vi "Jeffress_model_v004.vi"() -> ()   [LabVIEW 2019]
panel:
  out "Index":string
  out "new picture":picture
  in  "stop":bool
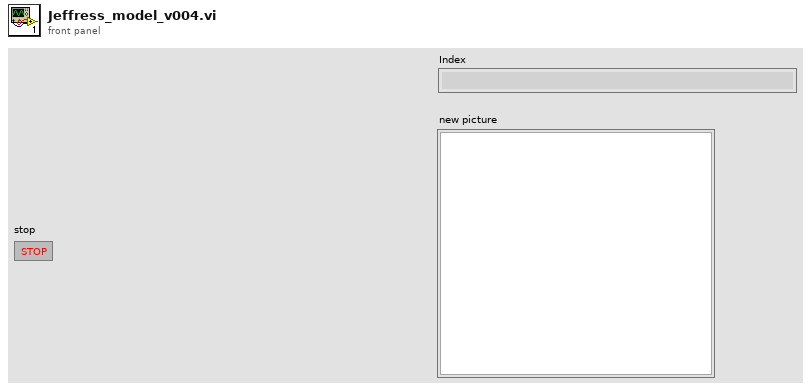
[diagram p1: front panel]
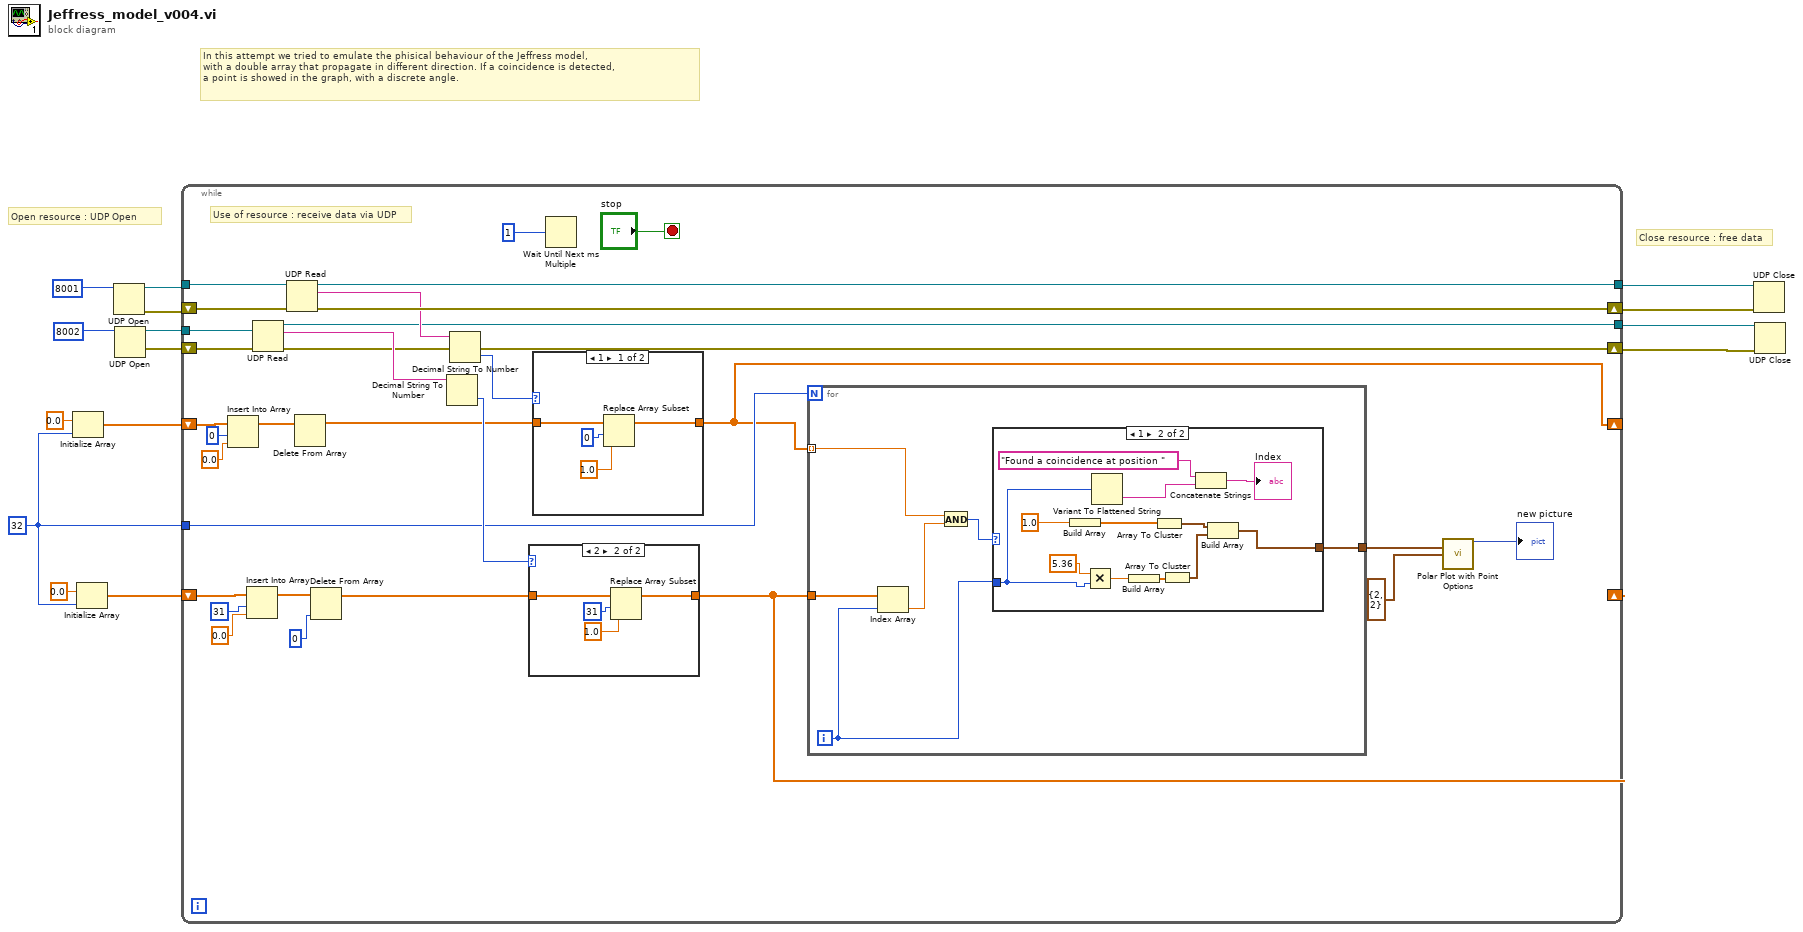
[diagram p0: block diagram]
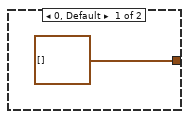
[diagram p2: hidden frame]
diagram:
  w1 = 32 ("dimension size")
  # "In this attempt we tried to emulate the phisical behaviour of the Jeffress model,\nwith a double array that propagate in different direction. If a coincidence is detected,\na point is showed in the graph, with a discrete angle."
  # "Close resource : free data"
  # "Open resource : UDP Open"
  n1 = Initialize Array(0.0 ("element"), w1) -> (w4:dbl[])
  n2 = Initialize Array(0.0 ("element"), w1) -> (w2:dbl[])
  n3 = UDP Open(11:u16 8001) -> (port=w13:refnum<k16>, 0:w15:errorcluster)  [unwired: 4 in, 1 out]
  n4 = UDP Open(11:u16 8002) -> (port=w9:refnum<k16>, 0:w8:errorcluster)  [unwired: 4 in, 1 out]
  n5 = while {
    tunnel: w13 -> [w42]
    tunnel: [w41] -> w12
    shift-right: [w44] -> w14
    shift-left: w15 -> [w43]
    tunnel: w9 -> [w35]
    shift-right: [w31] -> w7
    shift-left: w8 -> [w34]
    tunnel: [w32] -> w6
    shift-right: [w16] -> _
    shift-left: w4 -> [w30]
    shift-right: [w17] -> _
    shift-left: w2 -> [w22]
    tunnel: w1 -> [w19]
    stop <- "stop" stop-if-true
    # "Use of resource : receive data via UDP"
    n6 = Insert Into Array(array=w30, index=0, new element=0.0 ("new element/subarray")) -> (w27:dbl[])
    n7 = Insert Into Array(array=w22, index=31, new element=0.0 ("new element/subarray")) -> (w23:dbl[])
    n8 = UDP Read(connection ID=w35, 8:w34) -> (data out=w36:string, error out=w31:errorcluster, 3:w32:refnum<k16>)  [unwired: 2 in, 2 out]
    n9 = UDP Read(connection ID=w42, 8:w43) -> (data out=w37:string, error out=w44:errorcluster, 3:w41:refnum<k16>)  [unwired: 2 in, 2 out]
    n10 = Delete From Array(array=w27) -> (array with subset deleted=w26:dbl[])  [unwired: 2 in, 1 out]
    n11 = Delete From Array(array=w23, index=0) -> (array with subset deleted=w20:dbl[])  [unwired: 1 in, 1 out]
    n12 = Decimal String To Number(string=w36) -> (number=w33:i32)  [unwired: 2 in, 1 out]
    n13 = Decimal String To Number(string=w37) -> (number=w38:i32)  [unwired: 2 in, 1 out]
    n14 = case shown="2" w33 {
      tunnel: [w66 w68] -> w17
      tunnel: w20 -> [w66 w67]
      frame Default {
      }
      frame 2 {
        n15 = Replace Array Subset(array=w67, new element=1.0 ("new element/subarray"), index=31) -> (w68:dbl[])
      }
    }
    n16 = case shown="1" w38 {
      tunnel: [w72 w75] -> w16
      tunnel: w26 -> [w71 w75]
      frame 1 {
        n17 = Replace Array Subset(array=w71, new element=1.0 ("new element/subarray"), index=0) -> (w72:dbl[])
      }
      frame Default {
      }
    }
    n18 = Wait Until Next ms Multiple(millisecond multiple=u32 1) -> ()  [unwired: 1 out]
    n19 = for {
      N: w19 -> [_]
      tunnel: w16 -> [w50] mode=indexing
      tunnel: w17 -> [w52]
      tunnel: [w49] -> w18
      i -> [w47]
      n20 = Index Array(array=w52, index=w47) -> (element=w51:dbl)
      n21 = And(x=w50, y=w51) -> (x .and. y?=w48:i32)
      n22 = case shown="1" w48 {
        tunnel: w47 -> [_ w57]
        tunnel: [cluster{"magnitude":dbl, "phase":dbl}[] [] ("data array [mag, phase (deg)]") w58] -> w49
        frame 0, Default {
        }
        frame 1 {
          n23 = Build Array(1.0) -> (w62:dbl[])
          n24 = Multiply(x=5.36, y=w57) -> (x*y=w63:dbl)
          n25 = Variant To Flattened String(Variant=w57) -> (data string=w56:string)  [unwired: 1 out]
          n26 = Build Array(w63) -> (w61:dbl[])
          n27 = Array To Cluster(array=w62) -> (cluster=w60:cluster{"[0]":dbl, "[1]":dbl})
          n28 = Array To Cluster(array=w61) -> (cluster=w59:cluster{"[0]":dbl, "[1]":dbl})
          n29 = Concatenate Strings("Found a coincidence at position ", w56) -> (→"Index":string)
          n30 = Build Array(w60, w59) -> (w58:cluster{"[0]":dbl, "[1]":dbl}[])
        }
      }
    }
    n31 = call <vilib>:"Polar Plot with Point Options.vi"("data array [mag, phase (deg)]"=w18, "top left point(0, 0)"=cluster{"x":i16, "y":i16} {"x"=2, "y"=2}) -> ("new picture"=→"new picture":picture)  [unwired: 13 in]
  }
  n32 = UDP Close(connection ID=w12, 8:w14) -> ()  [unwired: 2 out]
  n33 = UDP Close(connection ID=w6, 8:w7) -> ()  [unwired: 2 out]
